vi "Resultados médios da norma.vi"(1 "IP":T1={"Diâmetro do furo [mm]"=1.4, "Diâmetro da linha média [mm]"=5.0, "Incremento de furação [mm]"=0.2, "Módulo de elasticidade [GPa]"=207.0, "Módulo de Poisson"=0.3, "Tipo de roseta utilizada"=enum."Tipo A", "Método de análise"=enum."Simplificado 2008"} caption="Infos para processamento", 2 "Dados in":T2) -> (0 "Resultados médios":string[][](array[string]))   [LabVIEW 2015]
uses:
  Controles/p,q, t, a e b.ctl
  Controles/Infos para processamento.ctl
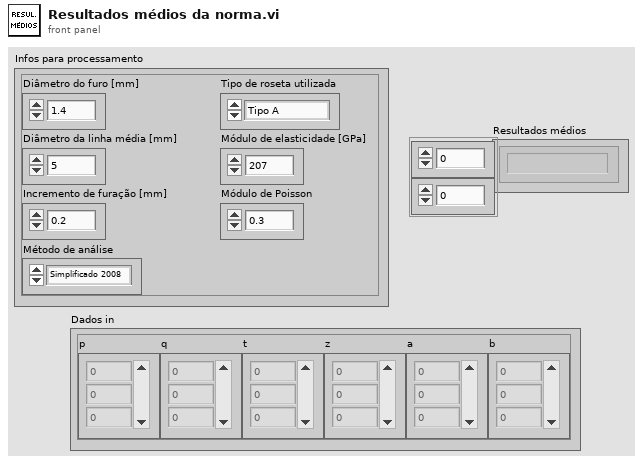
[diagram p1: front panel]
types:
  T1 = typedef "Infos para processamento.ctl" = cluster{"Diâmetro do furo [mm]":dbl, "Diâmetro da linha média [mm]":dbl, "Incremento de furação [mm]":dbl, "Módulo de elasticidade [GPa]":dbl, "Módulo de Poisson":dbl, "Tipo de roseta utilizada":enum16{"Tipo A", "Tipo B", "Tipo C"}, "Método de análise":enum16{"Não uniforme 2013", "Simplificado 2013", "Simplificado 2008"}}
  T2 = typedef "p,q, t, a e b.ctl" = cluster{"p":dbl[], "q":dbl[], "t":dbl[], "z":dbl[], "a":dbl[], "b":dbl[]}
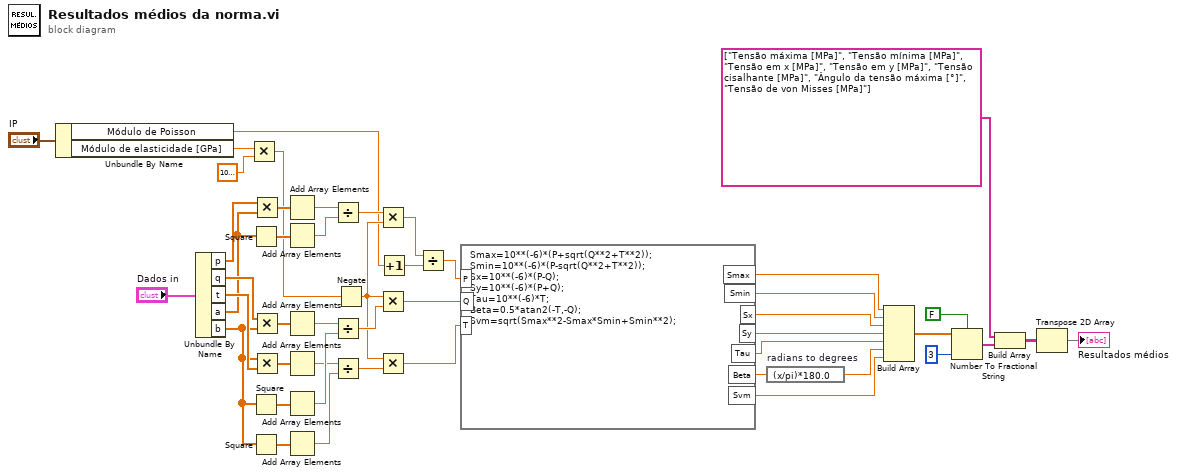
[diagram p0: block diagram]
diagram:
  n1 = Unbundle By Name("IP") -> ("Módulo de Poisson"=w2:dbl, "Módulo de elasticidade [GPa]"=w3:dbl)
  n2 = Unbundle By Name("Dados in") -> ("p"=w10:dbl[], "q"=w9:dbl[], "t"=w8:dbl[], "a"=w6:dbl[], "b"=w7:dbl[])
  n3 = Multiply(x=w3, y=1000000000.0) -> (x*y=w1:dbl)
  n4 = Square(x=w6) -> (x^2=w46:dbl[])
  n5 = Square(x=w7) -> (x^2=w38:dbl[])
  n6 = Square(x=w7) -> (x^2=w34:dbl[])
  n7 = Multiply(x=w10, y=w6) -> (x*y=w47:dbl[])
  n8 = Multiply(x=w9, y=w7) -> (x*y=w37:dbl[])
  n9 = Multiply(x=w7, y=w8) -> (x*y=w35:dbl[])
  n10 = Add Array Elements(numeric array=w47) -> (sum=w45:dbl)
  n11 = Add Array Elements(numeric array=w46) -> (sum=w44:dbl)
  n12 = Add Array Elements(numeric array=w37) -> (sum=w39:dbl)
  n13 = Add Array Elements(numeric array=w35) -> (sum=w33:dbl)
  n14 = Add Array Elements(numeric array=w38) -> (sum=w40:dbl)
  n15 = Add Array Elements(numeric array=w34) -> (sum=w32:dbl)
  n16 = Divide(x=w45, y=w44) -> (x/y=w43:dbl)
  n17 = Divide(x=w39, y=w40) -> (x/y=w36:dbl)
  n18 = Divide(x=w33, y=w32) -> (x/y=w30:dbl)
  n19 = Negate(x=w1) -> (-x=w31:dbl)
  n20 = Multiply(x=w43, y=w31) -> (x*y=w42:dbl)
  n21 = Multiply(x=w31, y=w36) -> (x*y=w28:dbl)
  n22 = Multiply(x=w31, y=w30) -> (x*y=w27:dbl)
  n23 = Increment(x=w2) -> (x+1=w41:dbl)
  n24 = Divide(x=w42, y=w41) -> (x/y=w29:dbl)
  n25 = formula code="Smax=10**(-6)*(P+sqrt(Q**2+T**2));\nSmin=10**(-6)*(P-sqrt(Q**2+T**2));\nSx=10**(-6)*(P-Q);\nSy=10**(-6)*(P+Q);\nTau=10**(-6)*T;\nBeta=0.5*atan2(-T,-Q);\nSvm=sqrt(Smax**2-Smax*Smin+Smin**2);"("P"=w29, "Q"=w28, "T"=w27) -> ("Smax"=w26:dbl, "Smin"=w25:dbl, "Sx"=w24:dbl, "Sy"=w23:dbl, "Tau"=w22:dbl, "Beta"=w13:dbl, "Svm"=w21:dbl)
  n26 = expression code="(x/pi)*180.0" "radians to degrees"(w13) -> (w12:dbl)
  n27 = Build Array(w26, w25, w24, w23, w22, w12, w21) -> (w20:dbl[])
  n28 = Number To Fractional String(use system decimal point (T)=FALSE, number=w20, precision (6)=i16 3) -> (F-format string=w17:string[])  [unwired: 1 in]
  n29 = Build Array(string[] ["Tensão máxima [MPa]", "Tensão mínima [MPa]", "Tensão em x [MPa]", "Tensão em y [MPa]", "Tensão cisalhante [MPa]", "Ângulo da tensão máxima [°]", "Tensão de von Misses [MPa]"] ("element"), w17) -> (w15:string[][])
  n30 = Transpose 2D Array(2D array=w15) -> (transposed array=→"Resultados médios":string[][])
